vi "Set Property.vi"(10 "Ctl Ref":refnum<vi>, 11 "UIP In":refnum<class "TemplateUIP.lvclass">) -> (0 "Error Out":errorcluster, 3 "UIP Out":refnum<class "TemplateUIP.lvclass">)   [LabVIEW 2015, in "TemplateUIP.lvclass"]
doc: "Modify this method to implement functionality for applying the UIP data to the property from VI Server Control."
uses:
  TemplateUIP.lvclass
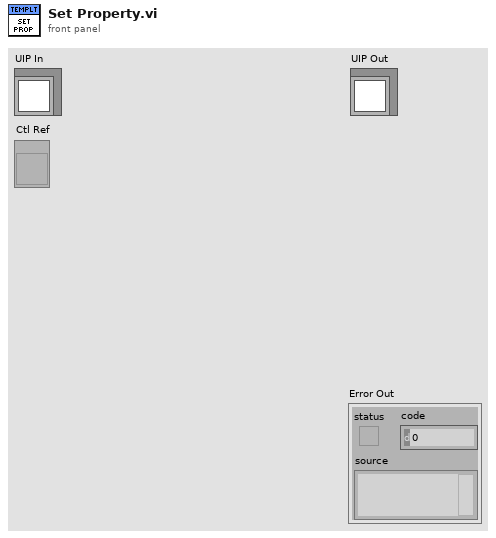
[diagram p1: front panel]
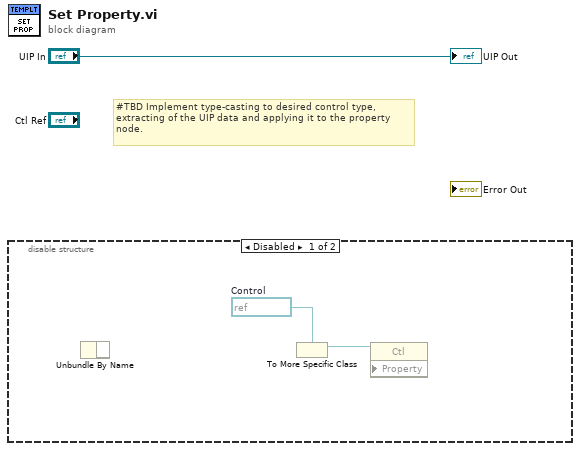
[diagram p0: block diagram]
diagram:
  # "#TBD Implement type-casting to desired control type,\nextracting of the UIP data and applying it to the property\nnode."
  n1 = disable-structure shown="Disabled" {
    frame Disabled {
      w3 = refnum<vi> refnum  # Control
      n2 = Unbundle By Name "Unbundle By Name"() -> ()  [unwired: 1 in, 1 out]
      n3 = To More Specific Class(target class=w3) -> (specific class reference=w2:refnum<vi>)  [unwired: 2 in, 1 out]
      n4 = property class="Ctl" props=[](reference=w2) -> ()  [unwired: 2 in, 2 out]
    }
    frame Enabled {
    }
  }
  "UIP Out" <- "UIP In"
